vi "Acc_Sorting.vi"(7 "withPreAccData":bool, 8 "error in":errorcluster, 9 "Percent":dbl=1.0, 10 "loadDataIn":dbl[][](array[numeric]), 11 "File path":path) -> (0 "error out":errorcluster, 2 "Test_Data":dbl[][](array[numeric]), 3 "file path Out":path)   [LabVIEW 2025]
uses:
  ee6ee51c-733a-4a27-9472-b61d3ffdaeb3.vi
  <vilib>/Array/Sort 2D Array - Pop Stack.vi
  <vilib>/Array/Sort 2D Array - Push Stack.vi
  ee6ee51c-733a-4a27-9472-b61d3ffdaeb3.vi/269d4b3b-47f5-49e3-8884-44851e4dd9d5.vi
  ee6ee51c-733a-4a27-9472-b61d3ffdaeb3.vi/6d99389c-673d-4efb-bf33-19b32bcf4cf8.vi
  <vilib>/Utility/file.llb/Read Delimited Spreadsheet (DBL).vi
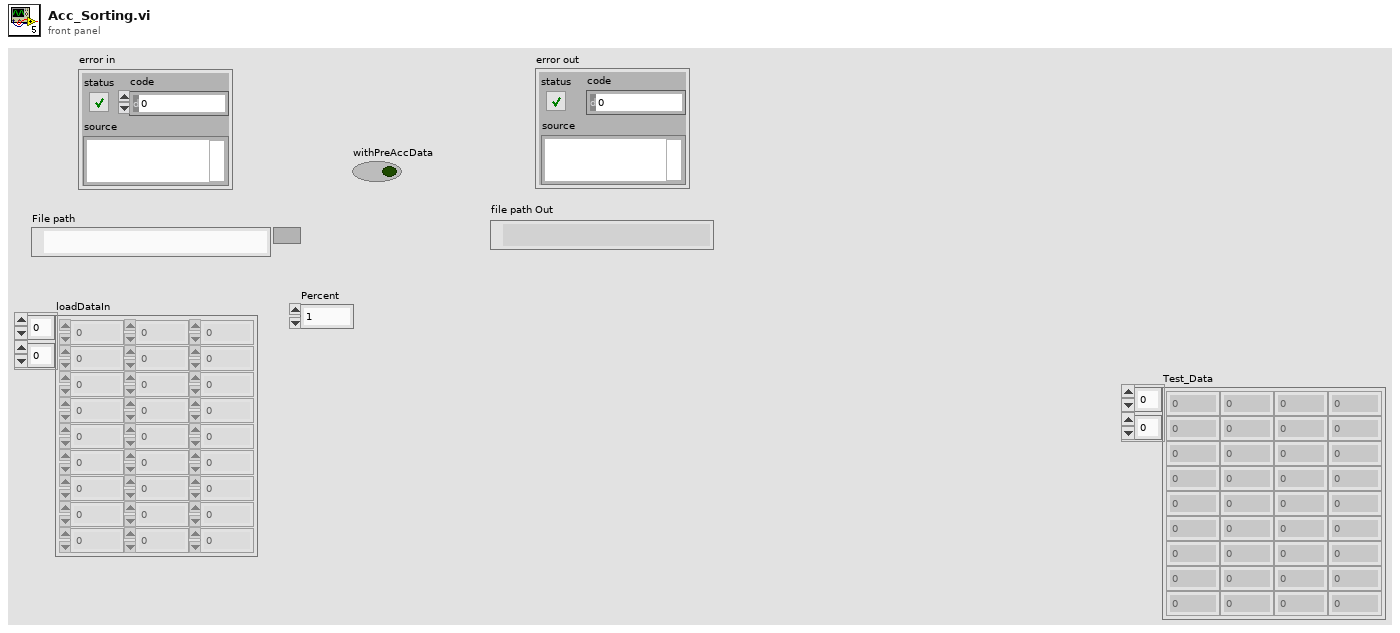
[diagram p1: front panel]
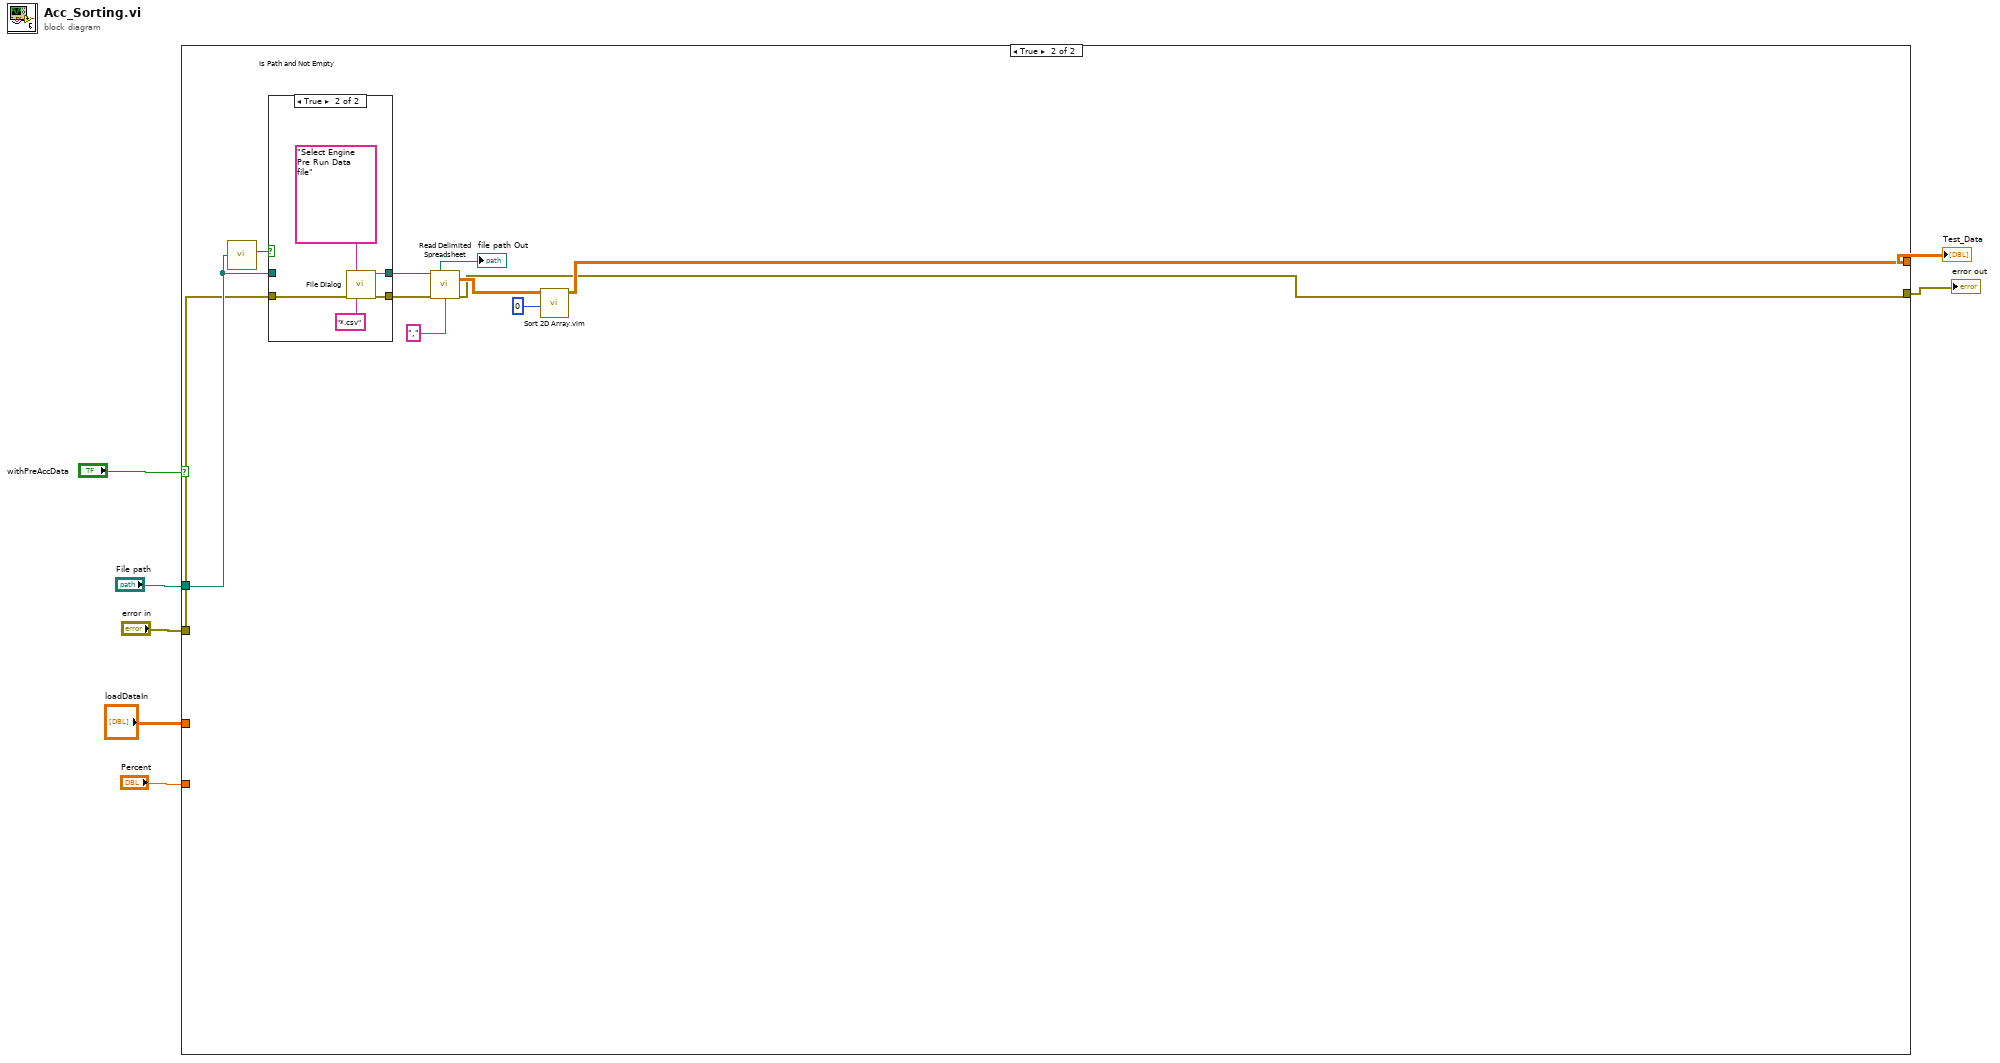
[diagram p0: block diagram]
diagram:
  n1 = case shown="True" "withPreAccData" {
    tunnel: [w8 w11] -> w7
    tunnel: "loadDataIn" -> [w8 _]
    tunnel: [w9 w10] -> w5
    tunnel: "File path" -> [_ w15]
    tunnel: "Percent" -> [_ _]
    tunnel: "error in" -> [w9 w13]
    frame False {
    }
    frame True {
      n2 = call <vilib>:"Is Path and Not Empty.vi"("path"=w15) -> ("Is Path and Not Empty?"=w17:bool)  [unwired: 4 in]
      n3 = case shown="True" w17 {
        tunnel: [w22 w27] -> w16
        tunnel: w15 -> [w22 _]
        tunnel: w13 -> [w21 w24]
        tunnel: [w21 w23] -> w12
        frame False {
        }
        frame True {
          n4 = call "File Dialog"("prompt"="Select Engine Pre Run Data file", "error in"=w24, "pattern (all files)"="*.csv") -> ("selected path"=w27:path, "error out"=w23:errorcluster)  [unwired: 9 in, 2 out]
        }
      }
      n5 = call-poly <vilib>:"Read Delimited Spreadsheet.vi"("file path (dialog if empty)"=w16, "error in (no error)"=w12, "delimiter (\\t)"="," ("delimiter (\\t)")) -> ("new file path (Not A Path if cancelled)"=→"file path Out":path, "all rows"=w19:dbl[][], "error out"=w10:errorcluster)  [unwired: 7 in, 3 out]
      n6 = call "Sort 2D Array.vim"("index"=0, "2D array"=w19) -> ("sorted 2D array"=w11:dbl[][])  [unwired: 8 in, 1 out]
    }
  }
  "Test_Data" <- w7
  "error out" <- w5
